vi "GetRFInjectedPwr.vi"(6 "Legacy (f)?":bool, 8 "error in (no error)":errorcluster, 10 "@ Frequency, MHz":dbl[](array[numeric])) -> (0 "error out":errorcluster, 2 "Injected Power, dBm":dbl[](array[numeric]))   [LabVIEW 2011]
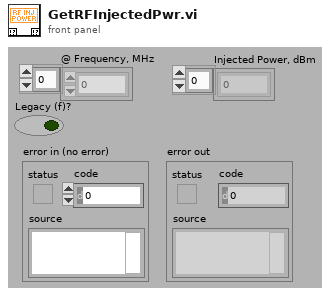
[diagram p1: front panel]
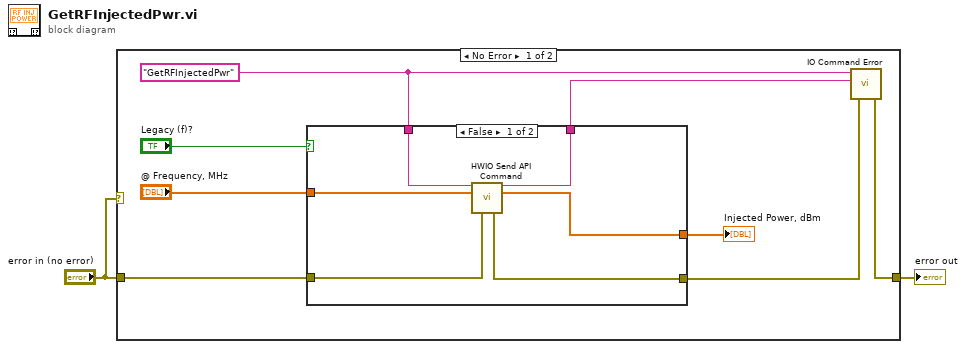
[diagram p0: block diagram]
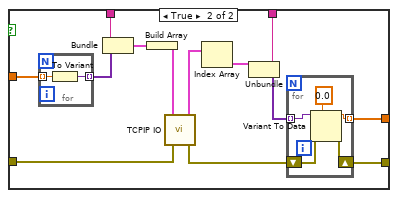
[diagram p2: hidden frame]
diagram:
  n1 = case shown="No Error" "error in (no error)" {
    tunnel: "error in (no error)" -> [w10 w37]
    tunnel: [w8 w37] -> w2
    frame No Error {
      w6 = "GetRFInjectedPwr"
      n2 = case shown="False" "Legacy (f)?" {
        tunnel: w10 -> [w14 w28]
        tunnel: [w13 w26] -> w9
        tunnel: [w15 w25] -> w7
        tunnel: w6 -> [w16 w24]
        tunnel: [w11 w20] -> w5
        tunnel: "@ Frequency, MHz" -> [w12 w18]
        frame False {
          n3 = call "HWIO Send API Command.vi"("Action"=w16, "Double"=w12, "error in (no error)"=w14) -> ("Action out"=w15:string, "Double out"=w11:dbl[], "error out"=w13:errorcluster)  [unwired: 5 in, 5 out]
        }
        frame True {
          n4 = for {
            tunnel: w18 -> [w31] mode=indexing
            tunnel: [w30] -> w17 mode=indexing
            n5 = To Variant(anything=w31) -> (Variant=w30:variant)
          }
          n6 = Bundle(w24, w17) -> (w29:cluster{string, variant[]})  [unwired: 1 out]
          n7 = Build Array(w29) -> (w21:cluster{string, variant[]}[])
          n8 = call "TCPIP IO.vi"("error in (no error)"=w28, "Commands"=w21) -> ("error out"=w27:errorcluster, "Responses"=w23:cluster{string, variant[]}[])  [unwired: 1 in, 3 out]
          n9 = Index Array(array=w23) -> (element=w22:cluster{string, variant[]})  [unwired: 1 in]
          n10 = Unbundle(w22) -> (w25:string, w19:variant[])
          n11 = for {
            tunnel: [w34] -> w20 mode=indexing
            shift-right: [w33] -> w26
            shift-left: w27 -> [w36]
            tunnel: w19 -> [w32] mode=indexing
            n12 = Variant To Data(error in=w36, type=0.0 ("Injected Power, dBm"), Variant=w32) -> (data=w34:dbl, error out=w33:errorcluster)
          }
        }
      }
      "Injected Power, dBm" <- w5
      n13 = call "IO Command Error.vi"("error in (no error)"=w9, "Command Returned (\"\")"=w7, "Command Sent (\"\")"=w6) -> ("error out"=w8:errorcluster)  [unwired: 4 out]
    }
    frame Error {
    }
  }
  "error out" <- w2
